vi "Configure Input Channels.vi"(8 "error in (no error)":errorcluster, 10 "Input Channel Refs":T1[](array[typedef]) format="%.0x", 11 "Device Ref in":T1 format="%.0x") -> (0 "error out":errorcluster, 1 "Input Channels":T4 {"Input Block Data Refs"."Data Reference" format="%.0x"}, 2 "RT FIFO Read out":refnum<k33>, 3 "Device Ref out":T1 format="%.0x")   [LabVIEW 2015, in "Shared Variable Custom Device.lvlib"]
doc: "Get the Input channels' block references and the RT FIFO Read."
uses:
  Shared Variable Custom Device.lvlib
  <vilib>/NI Veristand/Custom Device API/Custom Device Item Ref.ctl
  <vilib>/NI Veristand/Custom Device API/Block Data Reference.ctl
  <vilib>/NI Veristand/Custom Device API/Data Reference.ctl
  <vilib>/NI Veristand/Custom Device API/Data Access Type.ctl
  <vilib>/NI Veristand/Custom Device API/Custom Device API.lvlib
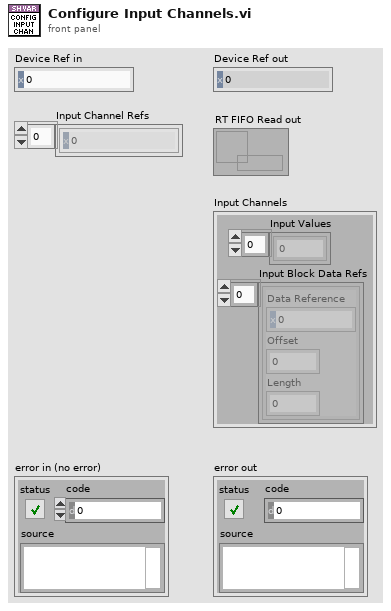
[diagram p1: front panel]
types:
  T1 = typedef "Custom Device API.lvlib/Custom Device Item Ref.ctl" = u64
  T2 = typedef "Custom Device API.lvlib/Block Data Reference.ctl" = cluster{"Data Reference":T3, "Offset":u64, "Length":u64}
  T3 = typedef "Custom Device API.lvlib/Data Reference.ctl" = i32
  T4 = cluster{"Input Values":dbl[], "Input Block Data Refs":T2[]}
  T5 = typedef "Custom Device API.lvlib/Data Access Type.ctl" = enum16{"Read", "Write"}
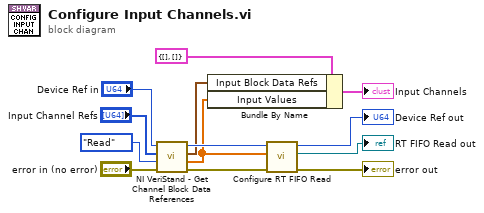
[diagram p0: block diagram]
diagram:
  n1 = call <vilib>:"NI VeriStand - Get Channel Block Data References.vi"("error in (no error)"="error in (no error)", "Access"=Data_Access_Type."Read", "Channel Refs"="Input Channel Refs", "Device Ref in"="Device Ref in") -> ("error out"=w10:errorcluster, "Values Array"=w5:dbl[], "Block Data Refs"=w6:T2[], "Device Ref out"=w9:T1)  [unwired: 4 in]
  n2 = Bundle By Name(cluster=T4 {"Input Values"=[], "Input Block Data Refs"=[]} ("Input Channels"), "Input Block Data Refs"=w6, "Input Values"=w5) -> (→"Input Channels":T4)
  n3 = call "Configure RT FIFO Read.vi"("error in (no error)"=w10, "Input Values Array"=w5, "Device Ref in"=w9) -> ("error out"=→"error out":errorcluster, "RT FIFO Read out"=→"RT FIFO Read out":refnum<k33>, "Device Ref out"=→"Device Ref out":T1)  [unwired: 6 in]
